vi "UVSC_DLL_path.vi"() -> ()   [LabVIEW 2011]
panel:
  in  "Path":path=path "UVSC.dll"
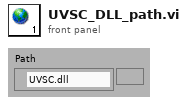
[diagram p1: front panel]
diagram:
